vi "uService GUI.vi"(8 "error in (no error)":errorcluster, 11 "uService Template in":refnum<class "TCP Writer.lvclass">) -> (3 "uService Template out":refnum<class "TCP Writer.lvclass">)   [LabVIEW 2026, in "TALOS.lvlib" / "TCP Writer.lvlib" / "TCP Writer.lvclass"]
uses:
  TCP Writer.lvclass
  C:/LabVIEW Code/TALOS/talos/Father of all uServices/Father of all uServices/Father of all uServices.lvclass
  Ancestor/Ancestor/Ancestor.lvclass/Ancestor.ctl
  Support VIs/Substitute Error.vi
  Support VIs/Generate Error.vi
  FGV/Error Memory/Get Error Description.vi
  Support VIs/Get PC name.vi
  Ancestor/Ancestor/Read ID.vi
  Support VIs/Get Class Name.vi
  FGV/Error Memory/Error Memory Core.vi
  <vilib>/AdvancedString/Delimited String to 1D String Array.vi
  <vilib>/AdvancedString/Delimited String to 1D String Array (string).vi
  Support VIs/Circus Root Path.vi
  FGV/Error Memory/Error Crt Lvl checker.vi
  FGV/Error Memory/Error Memory Core.vi/40c8088d-b597-4017-91af-faa98e00292e.vi
  FGV/Error Memory/Error Memory Core.vi/d4a3ab98-063c-4e44-b43d-fbdcfe6c2be2.vi
  Father of all uServices/Father of all uServices/Father of all uServices.lvclass
  C:/LabVIEW Code/TALOS/builds/Actor Framework PPL/Actor Framework.lvlibp/1abvi3w/vi.lib/ActorFramework/Actor/Actor.lvclass
  builds/Actor Framework PPL/Actor Framework.lvlibp/1abvi3w/vi.lib/ActorFramework/Actor/Read Self Enqueuer.vi
  builds/Actor Framework PPL/Actor Framework.lvlibp/1abvi3w/vi.lib/ActorFramework/Stop Msg/Send Normal Stop.vi
  Support VIs/Global Memory.vi
  <vilib>/Utility/LVClass/Get LV Class Name.vi
  Support VIs/Is in Packed Library.vi
  Support VIs/TALOS Root path.vi
  Support VIs/Read CSV worksheet.vi
  Support VIs/Global Constants.vi
  <vilib>/Utility/error.llb/General Error Handler.vi
  Support VIs/Error Log.vi
  Ancestor/Ancestor/Ancestor.lvclass
  <vilib>/Comparison/Equal/Equal Functor/Equal Functor.lvclass
panel:
  out "Textual":bool
  in  "Enable Output":bool
  out "TCP Writer Consumer Case":string
  out "TCP Writer Log":string
  in  "Send message":bool
  in  "Message":string
  in  "Recipient":string
  in  "Data":string
  out "Safe Mode":bool
  in  "Stop":bool
  out "uService ID":string
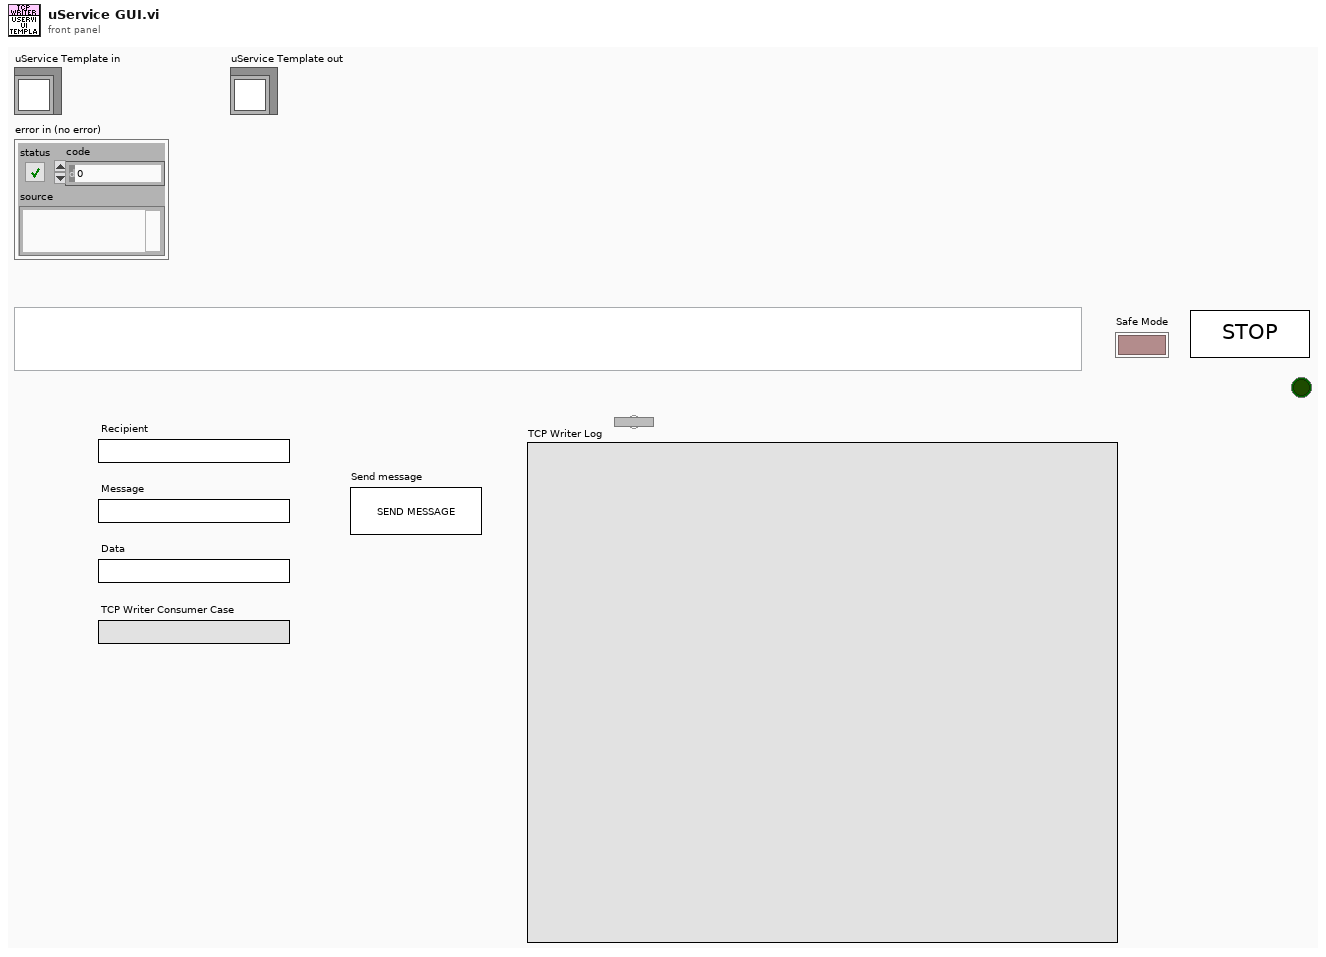
[diagram p1: front panel]
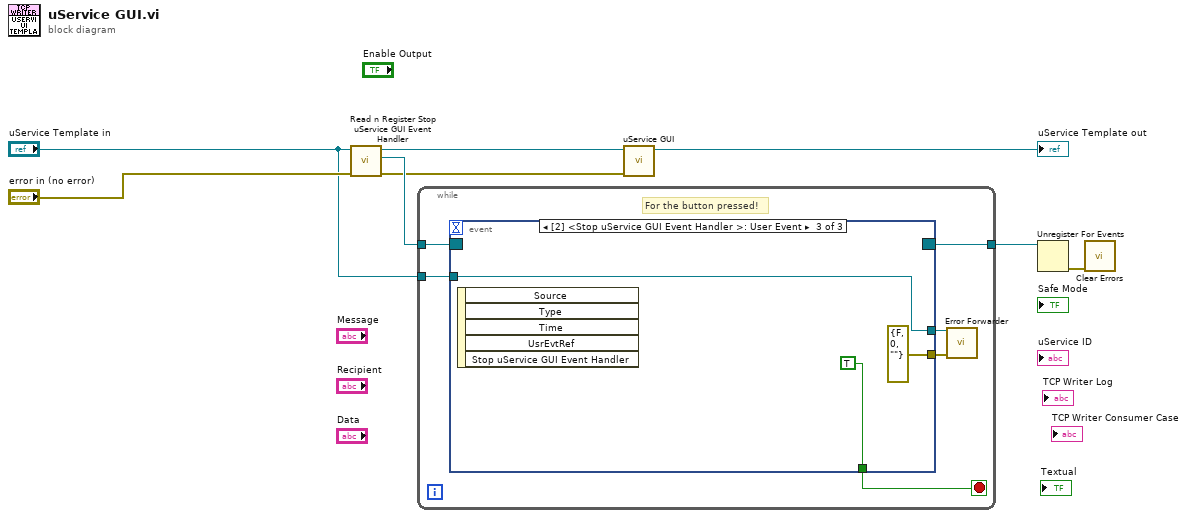
[diagram p0: block diagram]
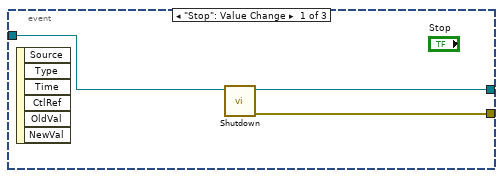
[diagram p2: hidden frame]
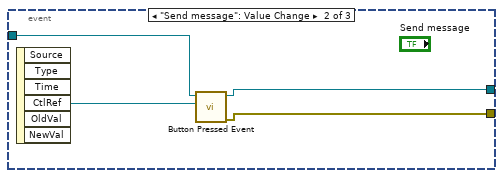
[diagram p3: hidden frame]
diagram:
  n1 = call-dynamic "Read n Register Stop uService GUI Event Handler .vi"("error in (no error)"="error in (no error)", "uService Template in"="uService Template in") -> ("error out"=w4:errorcluster, "Stop uService GUI Event Ref"=w6:refnum<event-registration>, "uService Template out"=w5:refnum<class "TCP Writer.lvclass">)  [unwired: 7 in]
  n2 = while {
    tunnel: [w14] -> w7
    tunnel: "uService Template in" -> [w12]
    tunnel: w6 -> [w11]
    stop <- w13 stop-if-true
    # "For the button pressed!"
    n3 = event shown="[2] <Stop uService GUI Event Handler >: User Event" {
      selector: w11 -> [_ _ _]
      dyn-events: [_ _ _] -> w14
      timeout: _ -> [_ _ _]
      tunnel: w12 -> [w17 w21 w23]
      tunnel: [_ _ TRUE] -> w13
      tunnel: [w16 w19 w23] -> w10
      tunnel: [w15 w18 errorcluster {"status"=FALSE, "code"=0, "source"=""} ("error out")] -> w9
      event "Stop": Value Change {
        n4 = event-data() -> ()  [unwired: 1 in, 6 out]
        n5 = call "Shutdown.vi"("Father of all uServices in"=w17) -> ("error out"=w15:errorcluster, "Father of all uServices out"=w16:refnum<class "TCP Writer.lvclass">)  [unwired: 9 in]
      }
      event "Send message": Value Change {
        n6 = event-data() -> ("CtlRef"=w20:refnum<vi>)  [unwired: 1 in, 5 out]
        n7 = call-dynamic "Button Pressed Event.vi"("CtlRef"=w20, "uService Template in"=w21) -> ("error out"=w18:errorcluster, "uService Template out"=w19:refnum<class "TCP Writer.lvclass">)  [unwired: 8 in]
      }
      event User Event {
        n8 = event-data() -> ()  [unwired: 1 in, 5 out]
      }
    }
    n9 = call "Error Forwarder.vi"("error in (no error)"=w9, "Father of all uServices in"=w10) -> ()  [unwired: 10 in]
  }
  n10 = call-parent "uService GUI.vi"("error in (no error)"=w4, "uService Template in"=w5) -> ("uService Template out"=→"uService Template out":refnum<class "TCP Writer.lvclass">)  [unwired: 9 in]
  n11 = Unregister For Events(event registration refnum=w7) -> (error out=w2:errorcluster)  [unwired: 1 in]
  n12 = call <vilib>:"Clear Errors.vi"("error in (no error)"=w2) -> ()  [unwired: 5 in, 2 out]
